vi "ETRONOutcountHourlyByMachine.vi"(7 "Machine":string="QAMT08", 8 "error in (no error) 2":errorcluster, 9 "report in":refnum<class "NI_report.lvclass">, 10 "error in (no error)":errorcluster, 11 "connection reference":T1) -> (0 "error in (no error) 3":errorcluster, 1 "report in 2":refnum<class "NI_report.lvclass">, 2 "error out":errorcluster, 3 "connection reference 2":T1)   [LabVIEW 2012]
uses:
  <vilib>/addons/database/Connection.llb/Conn ObjectReference.ctl
  <vilib>/Utility/NIReport.llb/NI_report.lvclass
  <vilib>/addons/database/Auxilliary.llb/DB Tools Cursor Type.ctl
  <vilib>/addons/database/Connection.llb/Conn Execute.vi
  <vilib>/addons/database/Recordset.llb/Rec Fetch Recordset Data (R).vi
  <vilib>/addons/database/Recordset.llb/Rec Destroy - Connection.vi
  <vilib>/addons/database/_DB Variant To Data/Database Variant To Data.xnode
  <vilib>/Utility/NIReport.llb/Excel/NI_Excel.lvclass
  <vilib>/addons/database/NI_Database_API.lvlib
panel:
  in  "?":cluster{"start row":i32, "start column":i32}
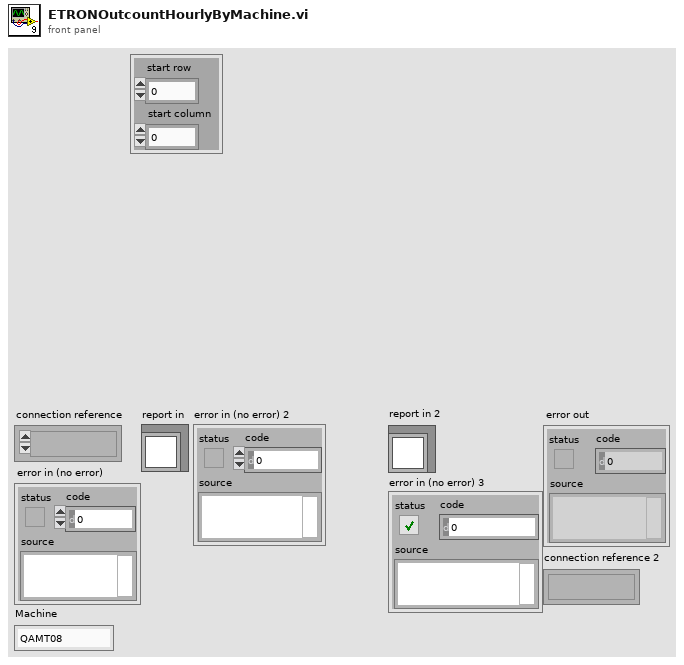
[diagram p1: front panel]
types:
  T1 = typedef "NI_Database_API.lvlib/Conn ObjectReference.ctl" = refnum<k1>
  T2 = typedef "NI_Database_API.lvlib/DB Tools Cursor Type.ctl" = enum16{"forward-only", "keyset", "dynamic", "static"}
  T3 = typedef "NI_Database_API.lvlib/Rec ObjectReference.ctl" = refnum<k1>
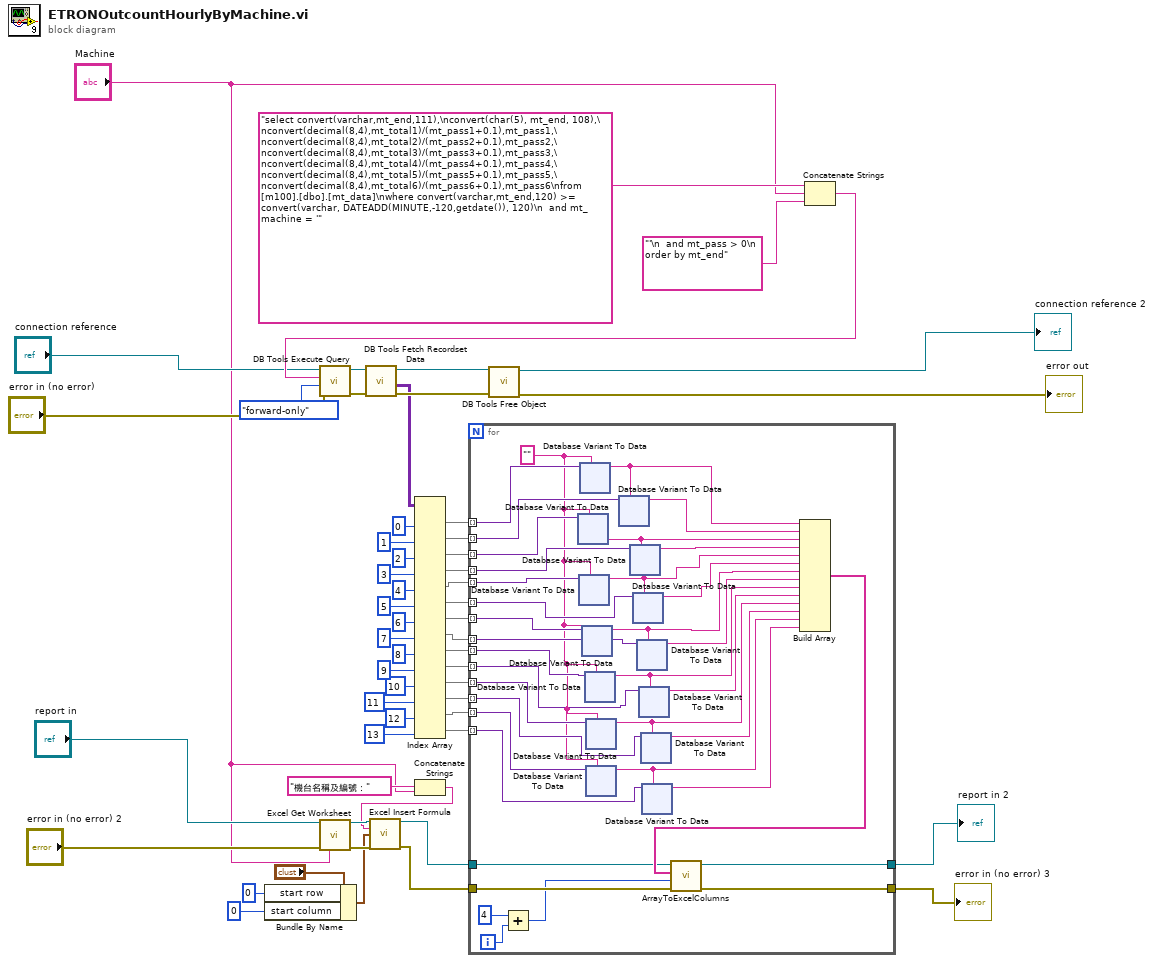
[diagram p0: block diagram]
diagram:
  n1 = Bundle By Name(cluster="?", "start row"=0, "start column"=0) -> (w14:cluster{"start row":i32, "start column":i32})
  n2 = call <vilib>:"Excel Get Worksheet.vi"("report in"="report in", "error in (no error)"="error in (no error) 2", "name (\"\")"="Machine") -> ("report out"=w19:refnum<class "NI_report.lvclass">, "error out"=w18:errorcluster)  [unwired: 11 in]
  n3 = Concatenate Strings("機台名稱及編號：" ("formula"), "Machine") -> (w11:string)
  n4 = call <vilib>:"Excel Insert Formula.vi"("report in"=w19, "formula"=w11, "start (0, 0)"=w14, "error in (no error)"=w18) -> ("report out"=w13:refnum<class "NI_report.lvclass">, "error out"=w12:errorcluster)  [unwired: 10 in]
  n5 = Concatenate Strings("select convert(varchar,mt_end,111),\nconvert(char(5), mt_end, 108),\nconvert(decimal(8,4),mt_total1)/(mt_pass1+0.1),mt_pass1,\nconvert(decimal(8,4),mt_total2)/(mt_pass2+0.1),mt_pass2,\nconvert(decimal(8,4),mt_total3)/(mt_pass3+0.1),mt_pass3,\nconvert(decimal(8,4),mt_total4)/(mt_pass4+0.1),mt_pass4,\nconvert(decimal(8,4),mt_total5)/(mt_pass5+0.1),mt_pass5,\nconvert(decimal(8,4),mt_total6)/(mt_pass6+0.1),mt_pass6\nfrom [m100].[dbo].[mt_data]\nwhere convert(varchar,mt_end,120) >=  convert(varchar, DATEADD(MINUTE,-120,getdate()), 120)\n  and mt_machine = '" ("SQL query"), "Machine", "'\n  and mt_pass > 0\n  order by mt_end" ("SQL query")) -> (w20:string)
  n6 = call-poly <vilib>:"DB Tools Execute Query.vi"("error in (no error)"="error in (no error)", "cursor type"=DB_Tools_Cursor_Type."forward-only", "SQL query"=w20, "connection reference"="connection reference") -> ("error out"=w56:errorcluster, "recordset reference"=w55:T3)  [unwired: 4 in]
  n7 = call-poly <vilib>:"DB Tools Fetch Recordset Data.vi"("error in (no error)"=w56, "recordset reference"=w55) -> ("error out"=w53:errorcluster, "recordset data"=w51:variant[][], "recordset reference out"=w54:T3)  [unwired: 3 in]
  n8 = Index Array(array=w51, index (col) #1=0 ("disabled index (col)"), index (col) #2=1 ("index (col)"), index (col) #3=2 ("index (col)"), index (col) #4=3 ("index (col)"), index (col) #5=4 ("index (col)"), index (col) #6=5 ("index (col)"), index (col) #7=6 ("index (col)"), index (col) #8=7 ("index (col)"), index (col) #9=8 ("index (col)"), index (col) #10=9 ("index (col)"), index (col) #11=10 ("index (col)"), index (col) #12=11 ("index (col)"), index (col) #13=12 ("index (col)"), index (col) #14=13 ("index (col)")) -> (element #1=w48:variant[], element #2=w47:variant[], element #3=w46:variant[], element #4=w35:variant[], element #5=w34:variant[], element #6=w33:variant[], element #7=w32:variant[], element #8=w31:variant[], element #9=w30:variant[], element #10=w29:variant[], element #11=w28:variant[], element #12=w27:variant[], element #13=w24:variant[], element #14=w23:variant[])  [unwired: 14 in]
  n9 = for {
    tunnel: w48 -> [w93] mode=indexing
    tunnel: w47 -> [w92] mode=indexing
    tunnel: w46 -> [w91] mode=indexing
    tunnel: w35 -> [w89] mode=indexing
    tunnel: w34 -> [w85] mode=indexing
    tunnel: w33 -> [w83] mode=indexing
    tunnel: w32 -> [w81] mode=indexing
    tunnel: w31 -> [w78] mode=indexing
    tunnel: w30 -> [w77] mode=indexing
    tunnel: w29 -> [w76] mode=indexing
    tunnel: w28 -> [w73] mode=indexing
    tunnel: w27 -> [w72] mode=indexing
    tunnel: w24 -> [w69] mode=indexing
    tunnel: w23 -> [w68] mode=indexing
    tunnel: w13 -> [w63]
    tunnel: w12 -> [w62]
    tunnel: [w58] -> w5
    tunnel: [w57] -> w4
    i -> [w61]
    w65 = ""
    n10 = Add(x=4, y=w61) -> (x+y=w59:i32)
    n11 = xnode "Database Variant To Data"("database variant"=w91, "type"=w65) -> ("data"=w87:string)  [unwired: 1 in, 1 out]
    n12 = xnode "Database Variant To Data"("database variant"=w85, "type"=w65) -> ("data"=w84:string)  [unwired: 1 in, 1 out]
    n13 = xnode "Database Variant To Data"("database variant"=w93, "type"=w65) -> ("data"=w88:string)  [unwired: 1 in, 1 out]
    n14 = xnode "Database Variant To Data"("database variant"=w81, "type"=w65) -> ("data"=w80:string)  [unwired: 1 in, 1 out]
    n15 = xnode "Database Variant To Data"("database variant"=w77, "type"=w65) -> ("data"=w75:string)  [unwired: 1 in, 1 out]
    n16 = xnode "Database Variant To Data"("database variant"=w73, "type"=w65) -> ("data"=w71:string)  [unwired: 1 in, 1 out]
    n17 = xnode "Database Variant To Data"("database variant"=w69, "type"=w65) -> ("data"=w67:string)  [unwired: 1 in, 1 out]
    n18 = xnode "Database Variant To Data"("database variant"=w92, "type"=w88) -> ("data"=w90:string)  [unwired: 1 in, 1 out]
    n19 = xnode "Database Variant To Data"("database variant"=w89, "type"=w87) -> ("data"=w86:string)  [unwired: 1 in, 1 out]
    n20 = xnode "Database Variant To Data"("database variant"=w83, "type"=w84) -> ("data"=w82:string)  [unwired: 1 in, 1 out]
    n21 = xnode "Database Variant To Data"("database variant"=w78, "type"=w80) -> ("data"=w79:string)  [unwired: 1 in, 1 out]
    n22 = xnode "Database Variant To Data"("database variant"=w76, "type"=w75) -> ("data"=w74:string)  [unwired: 1 in, 1 out]
    n23 = xnode "Database Variant To Data"("database variant"=w72, "type"=w71) -> ("data"=w70:string)  [unwired: 1 in, 1 out]
    n24 = xnode "Database Variant To Data"("database variant"=w68, "type"=w67) -> ("data"=w66:string)  [unwired: 1 in, 1 out]
    n25 = Build Array(w88, w90, w87, w86, w84, w82, w80, w79, w75, w74, w71, w70, w67, w66) -> (w64:string[])
    n26 = call "ArrayToExcelColumns.vi"("error in (no error)"=w62, "start row"=w59, "ArrayData"=w64, "report in"=w63) -> ("error in (no error) 2"=w57:errorcluster, "report in 2"=w58:refnum<class "NI_report.lvclass">)  [unwired: 6 in]
  }
  "report in 2" <- w5
  "error in (no error) 3" <- w4
  n27 = call-poly <vilib>:"DB Tools Free Object.vi"("error in (no error)"=w53, "recordset reference"=w54) -> ("error out"=→"error out":errorcluster, "connection reference"=→"connection reference 2":T1)  [unwired: 8 in]
